vi "enqueue.vi"(6 "priority (f)":bool, 8 "error in (no error)":errorcluster, 9 "data":errorcluster, 10 "states":T1, 11 "EventDaemon in":refnum<class "ErrorHandler.lvclass">) -> (0 "error out":errorcluster, 3 "EventDaemon out":refnum<class "ErrorHandler.lvclass">)   [LabVIEW 2024, in "ErrorHandler.lvclass"]
doc: "Enqueues private states for daemon. Set priority to True to enqueue to the front."
uses:
  ErrorHandler.lvclass
  ErrorHandler.lvclass/ErrorHandler.ctl
  states--enum.ctl
  msg--cluster.ctl
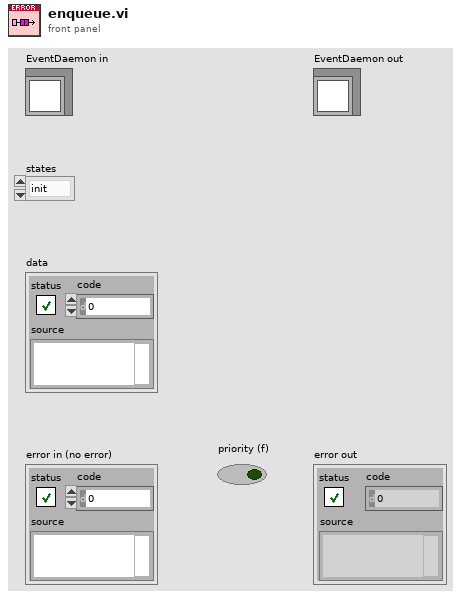
[diagram p1: front panel]
types:
  T1 = typedef "ErrorHandler.lvclass/states--enum.ctl" = enum16{"init", "default", "display error", "error handler", "exit"}
  T2 = typedef "ErrorHandler.lvclass/msg--cluster.ctl" = cluster{"cmd":T1, "error":errorcluster}
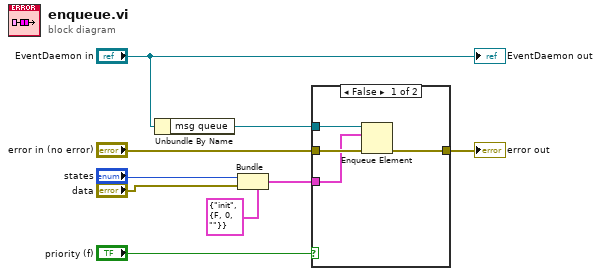
[diagram p0: block diagram]
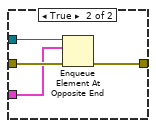
[diagram p2: hidden frame]
diagram:
  n1 = Unbundle By Name("EventDaemon in") -> ("msg queue"=w8:refnum<queue>)
  n2 = Bundle(cluster=T2 {"cmd"=enum."init", "error"={"status"=FALSE, "code"=0, "source"=""}} ("element"), "cmd"="states", "error"="data") -> (w1:T2)
  n3 = case shown="False" "priority (f)" {
    tunnel: w8 -> [w13 w17]
    tunnel: "error in (no error)" -> [w12 w16]
    tunnel: [w11 w15] -> w6
    tunnel: w1 -> [w10 w14]
    frame False {
      n4 = Enqueue Element(queue=w13, element=w10, error in (no error)=w12) -> (error out=w11:errorcluster)  [unwired: 1 in, 2 out]
    }
    frame True {
      n5 = Enqueue Element At Opposite End(queue=w17, element=w14, error in (no error)=w16) -> (error out=w15:errorcluster)  [unwired: 1 in, 2 out]
    }
  }
  "error out" <- w6
  "EventDaemon out" <- "EventDaemon in"
